vi "Apply EQ Correction.vi"(8 "gain correction (x/y)":dbl[](array[numeric]), 9 "frequency":dbl[](array[numeric]), 10 "amplitude":dbl, 11 "frequency":dbl) -> (3 "corrected amplitude":dbl)   [LabVIEW 2022 SP3]
uses:
  <vilib>/gmath/NI_Gmath.lvlib
panel:
  out "correction factor":dbl
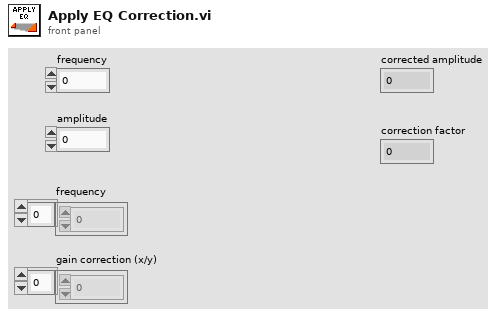
[diagram p1: front panel]
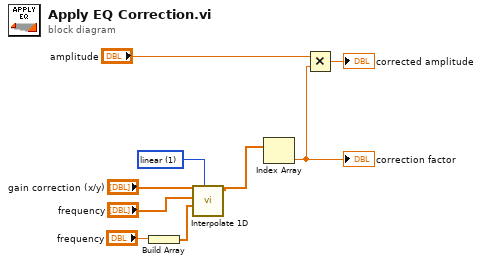
[diagram p0: block diagram]
diagram:
  w5 = 1 items=["nearest", "linear", "spline", "cubic Hermite", "Lagrange"] ("method")
  n1 = Build Array("frequency") -> (w6:dbl[])
  n2 = call <vilib>:"Interpolate 1D.vi"("method"=w5, "xi"=w6, "X"="frequency", "Y"="gain correction (x/y)") -> ("yi"=w4:dbl[])  [unwired: 5 in, 2 out]
  n3 = Index Array(array=w4) -> (element=w1:dbl)  [unwired: 1 in]
  "correction factor" <- w1
  n4 = Multiply(x="amplitude", y=w1) -> (x*y=→"corrected amplitude":dbl)
